vi "Logger_Clear.vi"(8 "error in (no error)":errorcluster, 11 "Logger Loop Cluster":T1={"Data Logger out"=refnum, "CAlexVersion"=enum."Mobile", "SyncIn"="", "SyncOut"=""}) -> (0 "error out":errorcluster)   [LabVIEW 2016]
uses:
  Logger Cluster.ctl
  Classes/DataLogger/Data Logger.lvclass
  Classes/CAlex2/TypeDef/CAlexVersion.ctl
  Classes/CAlex2/CAlex2.lvclass
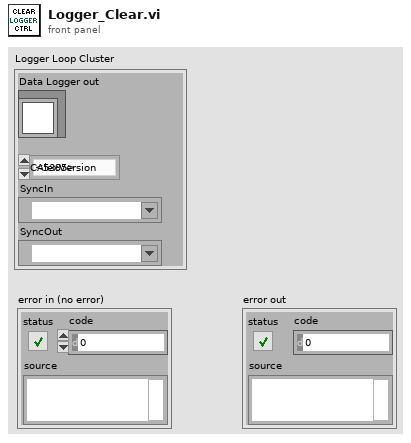
[diagram p1: front panel]
types:
  T1 = typedef "Logger Cluster.ctl" = cluster{"Data Logger out":refnum<class "Data Logger.lvclass">, "CAlexVersion":T2, "SyncIn":refnum<k21>, "SyncOut":refnum<k21>}
  T2 = typedef "CAlex2.lvclass/CAlexVersion.ctl" = enum16{"Bilateral", "Squat", "Bilateral_Squat", "Treadmill", "Mobile"}
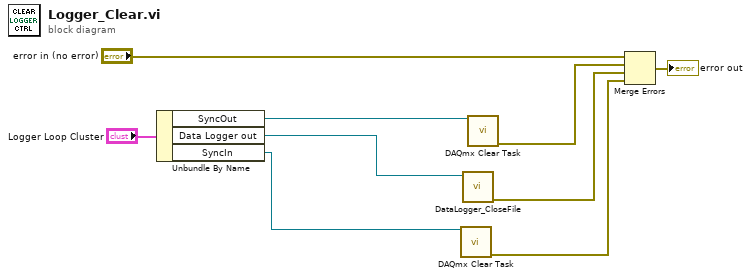
[diagram p0: block diagram]
diagram:
  n1 = Unbundle By Name("Logger Loop Cluster") -> ("SyncOut"=w8:refnum<k21>, "Data Logger out"=w7:refnum<class "Data Logger.lvclass">, "SyncIn"=w6:refnum<k21>)
  n2 = call <vilib>:"DAQmx Clear Task.vi"("task in"=w6) -> ("error out"=w5:errorcluster)  [unwired: 14 in]
  n3 = call "DataLogger_CloseFile.vi"("Data Logger in"=w7) -> ("error out"=w4:errorcluster)  [unwired: 9 in, 1 out]
  n4 = call <vilib>:"DAQmx Clear Task.vi"("task in"=w8) -> ("error out"=w3:errorcluster)  [unwired: 14 in]
  n5 = Merge Errors("error in (no error)", w3, w4, w5) -> (→"error out":errorcluster)
